vi "FTAnalyzer.vi"() -> ()   [LabVIEW 2014]
uses:
  <vilib>/Analysis/2dsp.llb/Real FFT.vi
  <vilib>/Analysis/NI_AALPro.lvlib
panel:
  in  "stop":bool
  in  "Time (s)":dbl
  in  "Rate":dbl
  in  "Averages":dbl
  out "FFT":dbl[](graph)
  out "Waveform Graph":waveform(dbl)(graph)
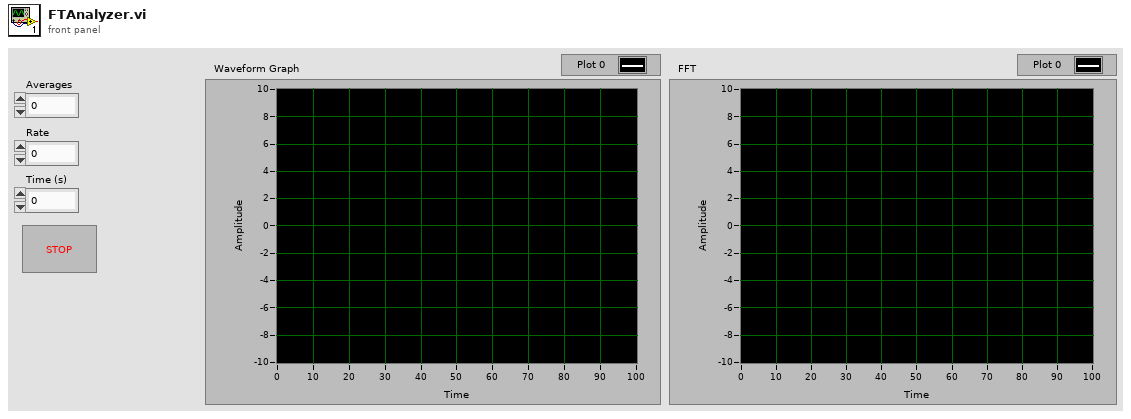
[diagram p1: front panel]
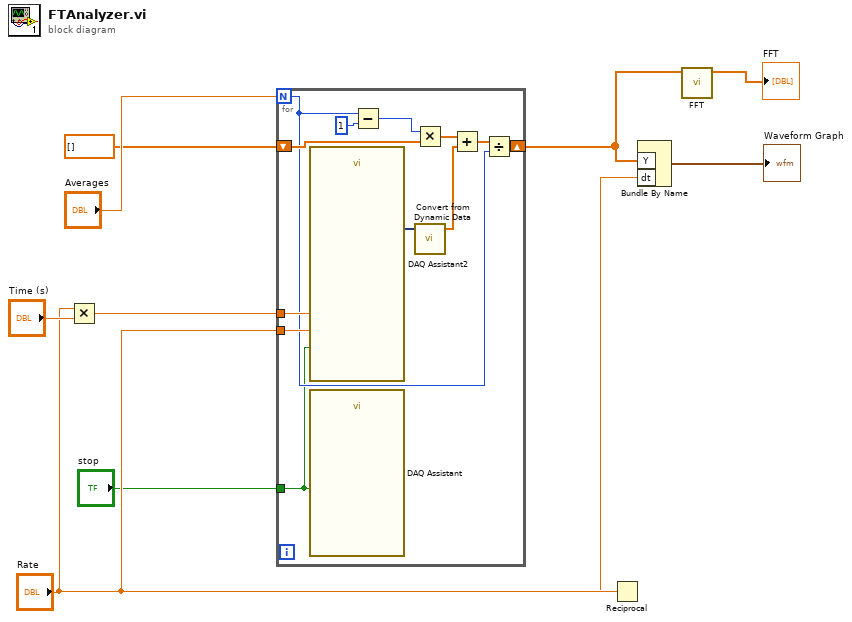
[diagram p0: block diagram]
diagram:
  n1 = Multiply(x="Rate", y="Time (s)") -> (x*y=w10:dbl)
  n2 = for {
    N: "Averages" -> [w13]
    tunnel: w10 -> [w22]
    tunnel: "Rate" -> [w21]
    shift-right: [w12] -> w3
    shift-left: dbl[] [] -> [w18]
    tunnel: "stop" -> [w11]
    n3 = call "DAQ Assistant2"("rate"=w21, "number of samples"=w22, "stop (T)"=w11) -> ("data"=w20:dynamicdata)  [unwired: 14 in, 2 out]
    n4 = call "DAQ Assistant"("stop (T)"=w11) -> ()  [unwired: 17 in, 2 out]
    n5 = Subtract(x=w13, y=1) -> (x-y=w16:i32)
    n6 = Multiply(x=w16, y=w18) -> (x*y=w15:dbl[])
    n7 = call "Convert from Dynamic Data"("Dynamic Data Type"=w20) -> ("Array"=w19:dbl[])  [unwired: 3 in]
    n8 = Add(x=w15, y=w19) -> (x+y=w14:dbl[])
    n9 = Divide(x=w14, y=w13) -> (x/y=w12:dbl[])
  }
  n10 = Reciprocal(x="Rate") -> (1/x=w5:dbl)
  n11 = Bundle By Name("Y"=w3, "dt"=w5) -> (→"Waveform Graph":waveform(dbl))  [unwired: 1 in]
  n12 = call-poly <vilib>:"FFT.vi"("X"=w3) -> ("FFT {X}"=→"FFT":cdb[])  [unwired: 9 in, 1 out]
